vi "Autonomous Independent.vi"() -> ()   [LabVIEW 2017]
doc: "This VI is called when autonomous begins, and will automatically be terminated when autonomous ends. You can carry out timed or sensor driven robot movement independently without needing to return to the caller."
uses:
  Public/Documents/Cross The Road Electronics/Phoenix-LabVIEW/Motor Controller/Controls/CTRE_Phoenix_MotorControl_ControlMode.ctl
  <vilib>/Rock Robotics/Network Tables/NT Read String.vi
  <vilib>/Rock Robotics/Network Tables/NT Read Number.vi
  <vilib>/Rock Robotics/Network Tables/NT Read Numeric Array.vi
  <vilib>/Rock Robotics/Network Tables/NT Read String Array.vi
  Robot Global Data.vi
  <vilib>/Rock Robotics/WPI/Ultrasonic/WPI_SonarMB1010AnalogRefNum Registry Get.vi
  <vilib>/Rock Robotics/WPI/Ultrasonic/WPI_SonarMB1010AnalogGetRange.vi
panel:
  out "Setpoint2":dbl
  out "Setpoint":dbl
  in  "Z Drive PID Gains":T1={"Position"=0.04, "Interval"=0.0, "Derivative"=0.0}
  # "Be sure to right-click and choose Data Operations>>Make Current Value default if you want to save the array values with the VI"
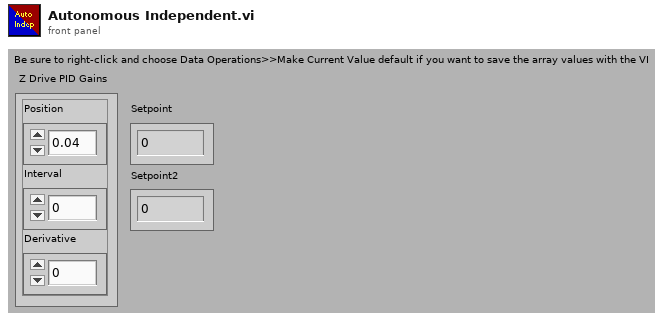
[diagram p1: front panel]
types:
  T1 = cluster{"Position":dbl, "Interval":dbl, "Derivative":dbl}
  T2 = enum16{"Front Left", "Front Right", "Back Left", "Back Right"}
  T3 = typedef "WPI_SonarMB1010AnalogDeviceRef.ctl" = cluster{"AIDeviceRef":T4, "Scaling factor (V/in)":dbl, "Average Bits":u8}
  T4 = typedef "WPI_AnalogChannelDevRef.ctl" = cluster{"DevStatus":errorcluster, "Analog Channel":T5}
  T5 = typedef "FPGA_AIChannel.ctl" = enum8{"AI 0", "AI 1", "AI 2", "AI 3", "AI MXP 0", "AI MXP 1", "AI MXP 2", "AI MXP 3", "Invalid"}
  T6 = typedef "WPI_AccelerometerDevRef.ctl" = cluster{"DevStatus":errorcluster, "Scaling":T7, "Analog Channels":T8, "I2C Bus":T9, "SPI Bus":T10, "Accel Range":T11, "ADXL Axes":T12, "Handle":i32, "Device Address":u8, "Accel Type":enum16{"Analog", "ADXL345 I2C", "ADXL345 SPI", "Internal", "ADXL362 SPI"}}
  T7 = typedef "WPI_AccelerometerScaling.ctl" = cluster{"Gain (VoltsPerG)":dbl, "Center Voltage":dbl}
  T8 = typedef "WPI_AccelerometerAnalogChannels.ctl" = cluster{"X-Axis":T5, "Y-Axis":T5, "Z-Axis":T5}
  T9 = typedef "i2c_bus.ctl" = enum16{"I2C On-Board", "I2C MXP", "Invalid"}
  T10 = typedef "spi_bus.ctl" = enum16{"SPI On-Board, CS0", "SPI On-Board, CS1", "SPI On-Board, CS2", "SPI On-Board, CS3", "SPI MXP", "Invalid"}
  T11 = typedef "ADXL345 Range.ctl" = u8
  T12 = typedef "WPI_AccelerometerADXL345 Axes.ctl" = cluster{"X-Axis":bool, "Y-Axis":bool, "Z-Axis":bool}
  T13 = cluster{"X-Axis":dbl, "Y-Axis":dbl, "Z-Axis":dbl}
  T14 = typedef "WPI_EncoderDevRef.ctl" = cluster{"DevStatus":errorcluster, "EncoderIndex":T15, "CounterIndex":T16, "DistancePerCount":dbl, "Decoding Type":T17}
  T15 = typedef "FPGA_EncoderIdx.ctl" = enum8{"Enc 0", "Enc 1", "Enc 2", "Enc 3", "Enc 4", "Enc 5", "Enc 6", "Enc 7", "Invalid"}
  T16 = typedef "FPGA_CounterCtrSystemIndex.ctl" = enum8{"Ctr 0", "Ctr 1", "Ctr 2", "Ctr 3", "Ctr 4", "Ctr 5", "Ctr 6", "Ctr 7", "Invalid"}
  T17 = typedef "WPI_EncoderType.ctl" = enum16{"1x", "2x", "4x"}
  T18 = typedef "WPI_MotorControlDeviceRef.ctl" = cluster{"DeviceStatus":errorcluster, "Type":T19, "PWM":cluster{"PWM Channel":T20, "DeadBand":T21}, "CAN":cluster{"Device Number":u8, "SetOutput VI Ref":variant, "GetOutput VI Ref":variant, "Enable VI Ref":variant, "Disable VI Ref":variant, "Data":variant}, "Invert":bool, "DIO PWM":cluster{"PWM \"Enable\" Channel":T20, "DIOChannel":T22, "PWM Rate":dbl}}
  T19 = typedef "WPI_MotorControlType.ctl" = enum16{"PWM", "CAN", "DIO PWM"}
  T20 = typedef "FPGA_DIOPWMChannel.ctl" = enum8{"PWM 0", "PWM 1", "PWM 2", "PWM 3", "PWM 4", "PWM 5", "PWM 6", "PWM 7", "PWM 8", "PWM 9", "PWM MXP 0", "PWM MXP 1", "PWM MXP 2", "PWM MXP 3", "PWM MXP 4", "PWM MXP 5", "PWM MXP 6", "PWM MXP 7", "PWM MXP 8", "PWM MXP 9", "Invalid"}
  T21 = typedef "WPI_PWMDeadband.ctl" = cluster{"Name":string, "maxPositivePwm":i32, "minPositivePwm":i32, "centerPwm":i32, "maxNegativePwm":i32, "minNegativePwm":i32, "angularRange":u16}
  T22 = typedef "FPGA_DIOChannel.ctl" = enum8{"DIO 0", "DIO 1", "DIO 2", "DIO 3", "DIO 4", "DIO 5", "DIO 6", "DIO 7", "DIO 8", "DIO 9", "DIO MXP 0", "DIO MXP 1", "DIO MXP 2", "DIO MXP 3", "DIO MXP 4", "DIO MXP 5", "DIO MXP 6", "DIO MXP 7", "DIO MXP 8", "DIO MXP 9", "DIO MXP 10", "DIO MXP 11", "DIO MXP 12", "DIO MXP 13", "DIO MXP 14", "DIO MXP 15", "SPI Port CS1", "SPI Port CS2", "SPI Port CS3", "SPI Port MISO", "SPI Port MOSI", "Invalid"}
  T23 = typedef "CTRE_Phoenix_MotorControl_ControlMode.ctl" = u16
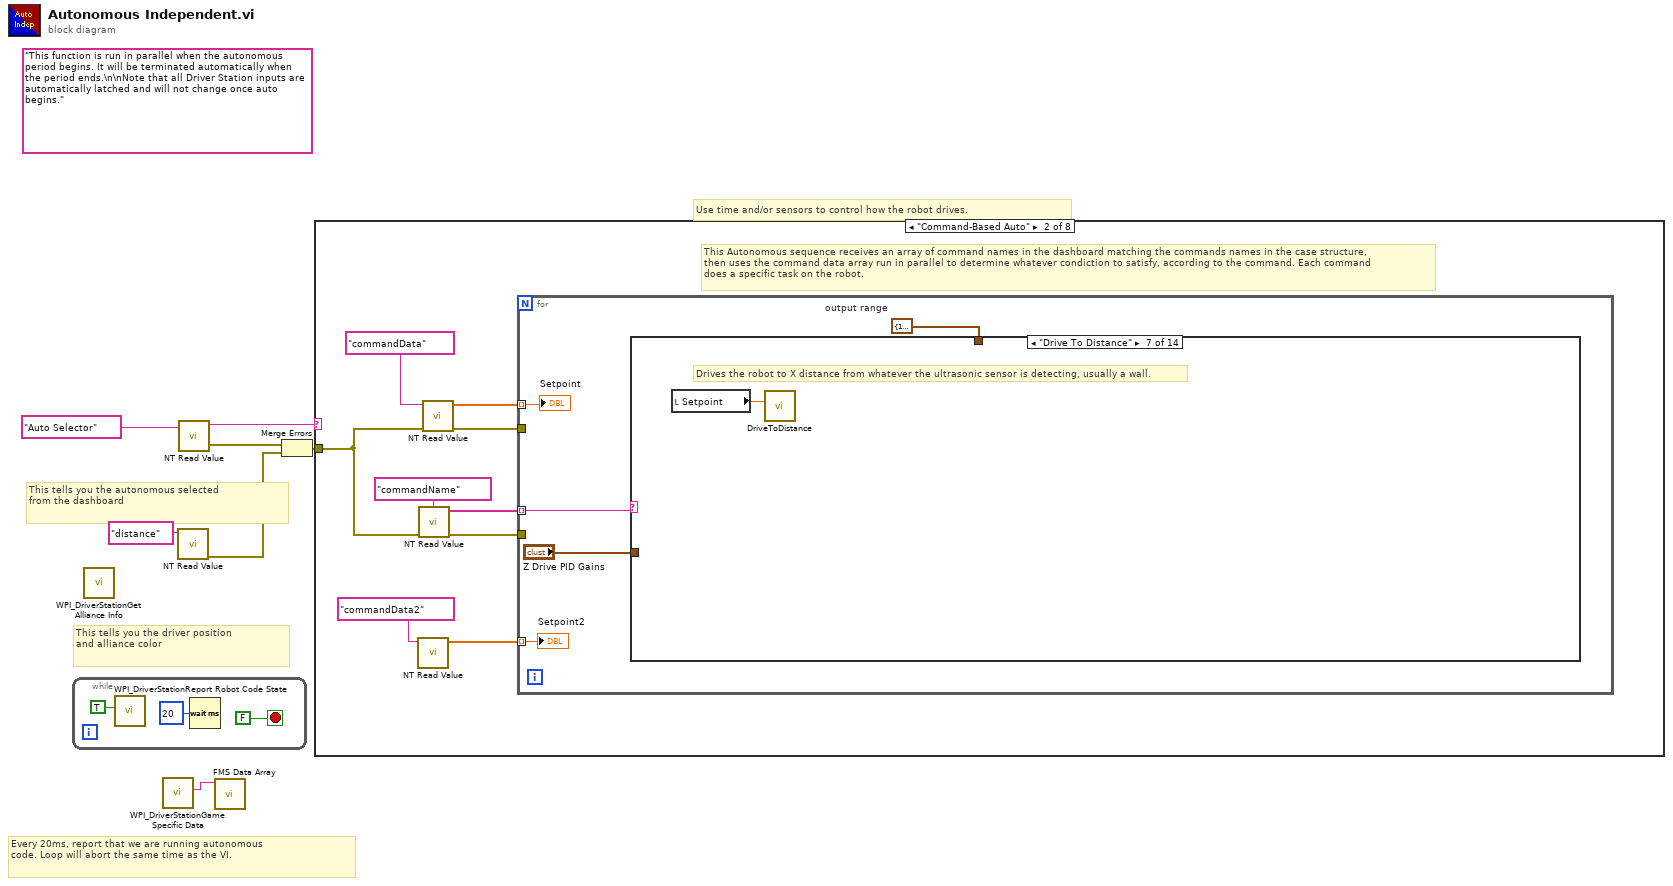
[diagram p0: block diagram]
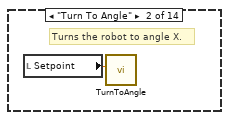
[diagram p4: hidden frame]
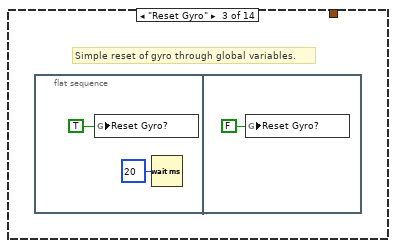
[diagram p5: hidden frame]
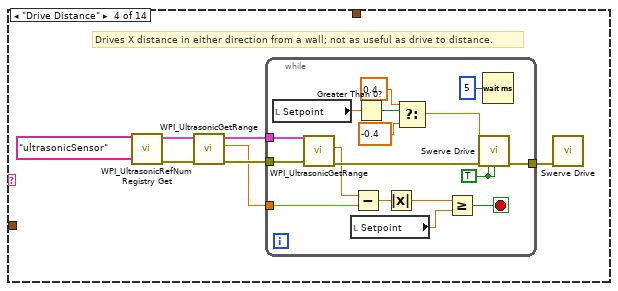
[diagram p6: hidden frame]
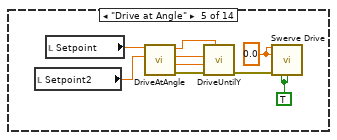
[diagram p7: hidden frame]
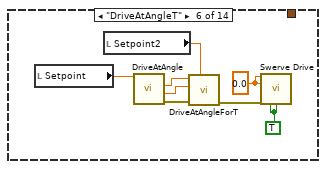
[diagram p8: hidden frame]
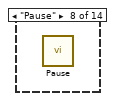
[diagram p9: hidden frame]
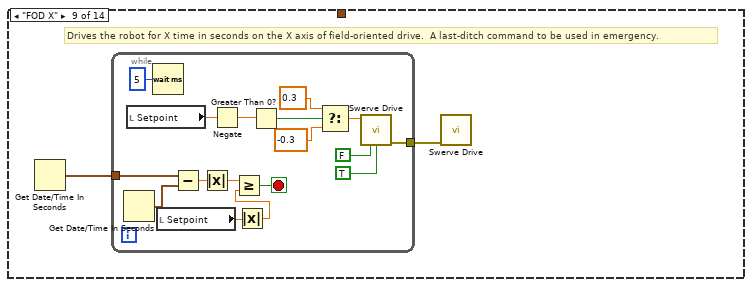
[diagram p10: hidden frame]
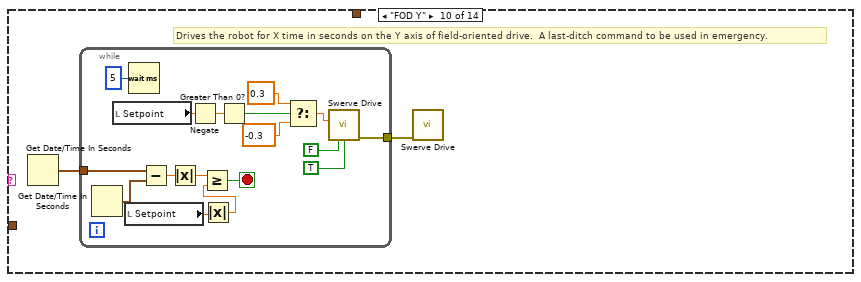
[diagram p11: hidden frame]
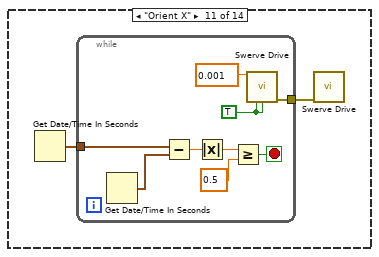
[diagram p12: hidden frame]
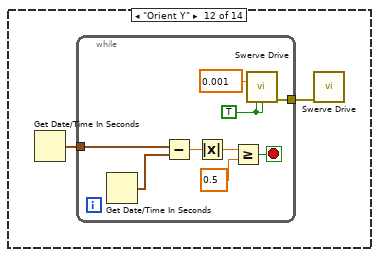
[diagram p13: hidden frame]
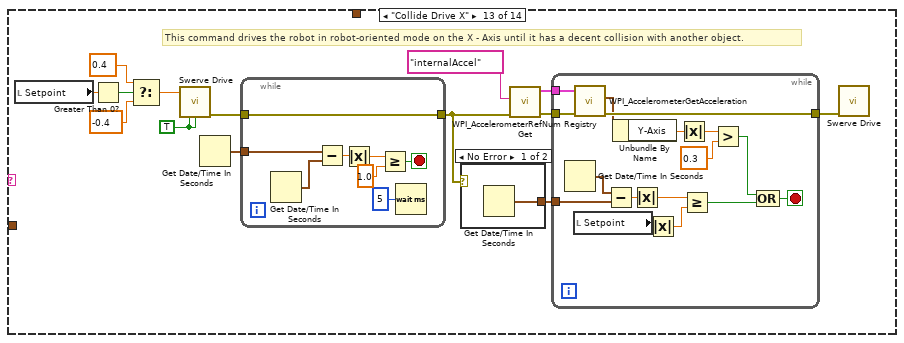
[diagram p14: hidden frame]
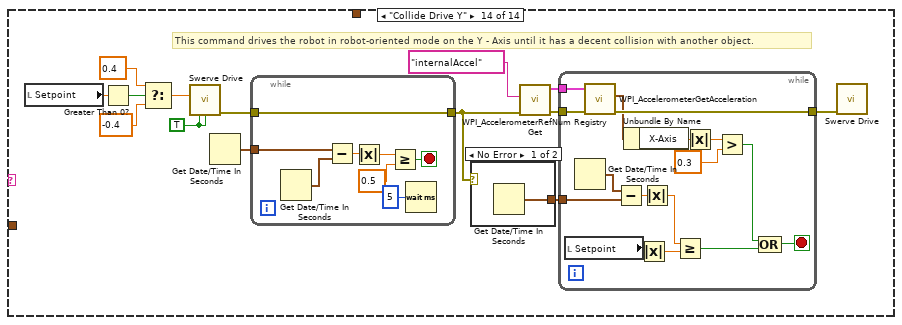
[diagram p16: hidden frame]
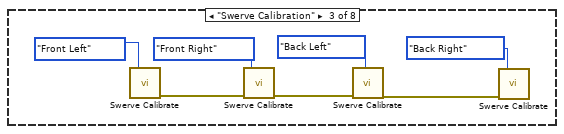
[diagram p18: hidden frame]
diagram:
  (unwired) "This function is run in parallel when the autonomous period begins. It will be terminated automatically when the period ends.\n\nNote that all Driver Station inputs are automatically latched and will not change once auto begins."
  # "This tells you the autonomous selected\nfrom the dashboard"
  # "Every 20ms, report that we are running autonomous\ncode. Loop will abort the same time as the VI."
  # "Use time and/or sensors to control how the robot drives."
  # "This tells you the driver position\nand alliance color"
  n1 = while {
    stop <- FALSE stop-if-true
    n2 = call <vilib>:"WPI_DriverStationReport Robot Code State.vi"("Autonomous"=TRUE) -> ()  [unwired: 10 in, 1 out]
    n3 = Wait (ms)(milliseconds to wait=u32 20) -> ()  [unwired: 1 out]
  }
  n4 = call <vilib>:"WPI_DriverStationGet Alliance Info.vi"() -> ()  [unwired: 12 out]
  n5 = call <vilib>:"WPI_DriverStationGame Specific Data.vi"() -> ("Game Specific Data"=w1:string)  [unwired: 11 in]
  n6 = call-poly <vilib>:"NT Read Value.vi"("Name"="distance") -> ("error out"=w3:errorcluster)  [unwired: 9 in, 1 out]
  n7 = call-poly <vilib>:"NT Read Value.vi"("Name"="Auto Selector") -> ("error out"=w4:errorcluster, "String"=w6:string)  [unwired: 9 in]
  n8 = call "FMS Data Array.vi"("Game Data"=w1) -> ()  [unwired: 8 in, 3 out]
  n9 = Merge Errors(w4, w3) -> (w2:errorcluster)
  n10 = case shown="\"Command-Based Auto\"" w6 {
    tunnel: w2 -> [_ w13 _ _ _ _ _ _]
    frame Default {
      # "You can put your main auto here, or you can right-click on the case and make any\nother frame be the default case."
      # "This is the frame that will execute if no selection is made, or if it is not recognized"
    }
    frame "Command-Based Auto" {
      # "This Autonomous sequence receives an array of command names in the dashboard matching the commands names in the case structure, \nthen uses the command data array run in parallel to determine whatever condiction to satisfy, according to the command. Each command\ndoes a specific task on the robot."
      n11 = call-poly <vilib>:"NT Read Value.vi"("Name"="commandData2") -> ("Numeric Array"=w11:dbl[])  [unwired: 9 in, 1 out]
      n12 = call-poly <vilib>:"NT Read Value.vi"("error in"=w13, "Name"="commandName") -> ("error out"=w14:errorcluster, "String Array"=w17:string[])  [unwired: 8 in]
      n13 = call-poly <vilib>:"NT Read Value.vi"("error in"=w13, "Name"="commandData") -> ("error out"=w15:errorcluster, "Numeric Array"=w16:dbl[])  [unwired: 8 in]
      n14 = for {
        tunnel: w17 -> [w24] mode=indexing
        tunnel: w16 -> [w21] mode=indexing
        tunnel: w15 -> [_]
        tunnel: w14 -> [_]
        tunnel: w11 -> [w20] mode=indexing
        w22 = cluster{"output high":dbl, "output low":dbl} {"output high"=1.0, "output low"=-1.0}  # output range
        n15 = case shown="\"Drive To Distance\"" w24 {
          tunnel: "Z Drive PID Gains" -> [_ _ _ _ _ _ _ _ _ _ _ _ _ _]
          tunnel: w22 -> [_ _ _ _ _ _ _ _ _ _ _ _ _ _]
          frame Default {
          }
          frame "Turn To Angle" {
            # "Turns the robot to angle X."
            n16 = local read "Setpoint"() -> (w25:dbl)
            n17 = call "TurnToAngle.vi"("Target Angle"=w25) -> ()  [unwired: 10 in, 1 out]
          }
          frame "Reset Gyro" {
            # "Simple reset of gyro through global variables."
            n18 = flat-sequence {
              frame #0 {
                n19 = global write "Robot Global Data.vi" "Reset Gyro?"(TRUE ("Reset Gyro?")) -> ()
                n20 = Wait (ms)(milliseconds to wait=u32 20) -> ()  [unwired: 1 out]
              }
              frame #1 {
                n21 = global write "Robot Global Data.vi" "Reset Gyro?"(FALSE ("Reset Gyro?")) -> ()
              }
            }
          }
          frame "Drive Distance" {
            # "Drives X distance in either direction from a wall; not as useful as drive to distance."
            n22 = call-poly <vilib>:"WPI_UltrasonicRefNum Registry Get.vi"("refnum name"="ultrasonicSensor") -> ("error out"=w31:errorcluster, "SonarMB1010AnalogDevRef"=w33:T3)  [unwired: 9 in]
            n23 = call-poly <vilib>:"WPI_UltrasonicGetRange.vi"("error in"=w31, "SonarMB1010AnalogDevRef"=w33) -> ("error out"=w30:errorcluster, "Distance"=w29:dbl, "SonarMB1010AnalogDevRef"=w32:T3)  [unwired: 7 in]
            n24 = while {
              tunnel: [w51] -> w34
              tunnel: w29 -> [w46]
              tunnel: w32 -> [w49]
              tunnel: w30 -> [w48]
              stop <- w50 stop-if-true
              w41 = TRUE ("Robot Centric?")
              n25 = local read "Setpoint"() -> (w39:dbl)
              n26 = call-poly <vilib>:"WPI_UltrasonicGetRange.vi"("error in"=w48, "SonarMB1010AnalogDevRef"=w49) -> ("error out"=w47:errorcluster, "Distance"=w40:dbl)  [unwired: 7 in, 1 out]
              n27 = local read "Setpoint"() -> (w38:dbl)
              n28 = Subtract(x=w40, y=w46) -> (x-y=w37:dbl)
              n29 = Greater Than 0?(x=w39) -> (x > 0?=w42:bool)
              n30 = Absolute Value(x=w37) -> (abs(x)=w52:dbl)
              n31 = Select(t=0.4 ("Y"), s=w42, f=-0.4 ("Y")) -> (s? t:f=w45:dbl)
              n32 = Greater Or Equal?(x=w52, y=w38) -> (x >= y?=w50:bool)
              n33 = call "Swerve Drive.vi"("Y"=w45, "Error In"=w47, "Robot Centric?"=w41, "Autonomous?"=w41) -> ("Error Out"=w51:errorcluster)  [unwired: 7 in, 4 out]
              n34 = Wait (ms)(milliseconds to wait=u32 5) -> ()  [unwired: 1 out]
            }
            n35 = call "Swerve Drive.vi"("Error In"=w34) -> ()  [unwired: 10 in, 5 out]
          }
          frame "Drive at Angle" {
            w56 = TRUE ("Autonomous?")
            w57 = 0.0
            n36 = local read "Setpoint2"() -> (w53:dbl)
            n37 = local read "Setpoint"() -> (w54:dbl)
            n38 = call "DriveAtAngle.vi"("Target Angle"=w54, "Distance"=w53) -> ("y-axis distance"=w55:dbl, "x"=w59:dbl, "y"=w58:dbl, "Error Out"=w60:errorcluster)  [unwired: 5 in]
            n39 = call "DriveUntilY.vi"("Ultrasonic Stop"=w55, "error in"=w60, "y"=w58, "x"=w59) -> ("error out"=w61:errorcluster)  [unwired: 7 in]
            n40 = call "Swerve Drive.vi"("X"=w57, "Y"=w57, "Error In"=w61, "Robot Centric?"=w56, "Autonomous?"=w56) -> ()  [unwired: 6 in, 5 out]
          }
          frame "DriveAtAngleT" {
            w67 = TRUE ("Autonomous?")
            w68 = 0.0
            n41 = local read "Setpoint"() -> (w69:dbl)
            n42 = local read "Setpoint2"() -> (w62:dbl)
            n43 = call "DriveAtAngle.vi"("Target Angle"=w69) -> ("x"=w66:dbl, "y"=w65:dbl, "Error Out"=w64:errorcluster)  [unwired: 6 in, 1 out]
            n44 = call "DriveAtAngleForT.vi"("time(sec)"=w62, "Error In"=w64, "y"=w65, "x"=w66) -> ("Error Out"=w63:errorcluster)  [unwired: 7 in]
            n45 = call "Swerve Drive.vi"("X"=w68, "Y"=w68, "Error In"=w63, "Robot Centric?"=w67, "Autonomous?"=w67) -> ()  [unwired: 6 in, 5 out]
          }
          frame "Drive To Distance" {
            # "Drives the robot to X distance from whatever the ultrasonic sensor is detecting, usually a wall."
            n46 = local read "Setpoint"() -> (w70:dbl)
            n47 = call "DriveToDistance.vi"("Setpoint"=w70) -> ()  [unwired: 10 in, 1 out]
          }
          frame "Pause" {
            n48 = call "Pause.vi"() -> ()  [unwired: 11 in, 1 out]
          }
          frame "FOD X" {
            # "Drives the robot for X time in seconds on the X axis of field-oriented drive.  A last-ditch command to be used in emergency."
            n49 = Get Date/Time In Seconds() -> (seconds since 1Jan1904=w72:timestamp)
            n50 = while {
              tunnel: w72 -> [w89]
              tunnel: [w83] -> w71
              stop <- w84 stop-if-true
              n51 = Get Date/Time In Seconds() -> (seconds since 1Jan1904=w88:timestamp)
              n52 = local read "Setpoint"() -> (w76:dbl)
              n53 = Wait (ms)(milliseconds to wait=u32 5) -> ()  [unwired: 1 out]
              n54 = local read "Setpoint"() -> (w85:dbl)
              n55 = Subtract(x=w89, y=w88) -> (x-y=w87:dbl)
              n56 = Absolute Value(x=w87) -> (abs(x)=w86:dbl)
              n57 = Negate(x=w76) -> (-x=w73:dbl)
              n58 = Absolute Value(x=w85) -> (abs(x)=w74:dbl)
              n59 = Greater Or Equal?(x=w86, y=w74) -> (x >= y?=w84:bool)
              n60 = Greater Than 0?(x=w73) -> (x > 0?=w77:bool)
              n61 = Select(t=0.3 ("X"), s=w77, f=-0.3 ("X")) -> (s? t:f=w78:dbl)
              n62 = call "Swerve Drive.vi"("X"=w78, "Robot Centric?"=FALSE, "Autonomous?"=TRUE) -> ("Error Out"=w83:errorcluster)  [unwired: 8 in, 4 out]
            }
            n63 = call "Swerve Drive.vi"("Error In"=w71) -> ()  [unwired: 10 in, 5 out]
          }
          frame "FOD Y" {
            # "Drives the robot for X time in seconds on the Y axis of field-oriented drive.  A last-ditch command to be used in emergency."
            n64 = Get Date/Time In Seconds() -> (seconds since 1Jan1904=w91:timestamp)
            n65 = while {
              tunnel: w91 -> [w108]
              tunnel: [w102] -> w90
              stop <- w103 stop-if-true
              n66 = Get Date/Time In Seconds() -> (seconds since 1Jan1904=w107:timestamp)
              n67 = local read "Setpoint"() -> (w95:dbl)
              n68 = local read "Setpoint"() -> (w104:dbl)
              n69 = Wait (ms)(milliseconds to wait=u32 5) -> ()  [unwired: 1 out]
              n70 = Subtract(x=w108, y=w107) -> (x-y=w106:dbl)
              n71 = Absolute Value(x=w106) -> (abs(x)=w105:dbl)
              n72 = Negate(x=w95) -> (-x=w92:dbl)
              n73 = Absolute Value(x=w104) -> (abs(x)=w93:dbl)
              n74 = Greater Or Equal?(x=w105, y=w93) -> (x >= y?=w103:bool)
              n75 = Greater Than 0?(x=w92) -> (x > 0?=w97:bool)
              n76 = Select(t=0.3 ("X"), s=w97, f=-0.3 ("X")) -> (s? t:f=w96:dbl)
              n77 = call "Swerve Drive.vi"("Y"=w96, "Robot Centric?"=FALSE, "Autonomous?"=TRUE) -> ("Error Out"=w102:errorcluster)  [unwired: 8 in, 4 out]
            }
            n78 = call "Swerve Drive.vi"("Error In"=w90) -> ()  [unwired: 10 in, 5 out]
          }
          frame "Orient X" {
            n79 = Get Date/Time In Seconds() -> (seconds since 1Jan1904=w110:timestamp)
            n80 = while {
              tunnel: w110 -> [w119]
              tunnel: [w113] -> w109
              stop <- w112 stop-if-true
              w114 = TRUE ("Robot Centric?")
              n81 = Get Date/Time In Seconds() -> (seconds since 1Jan1904=w118:timestamp)
              n82 = Subtract(x=w119, y=w118) -> (x-y=w117:dbl)
              n83 = Absolute Value(x=w117) -> (abs(x)=w116:dbl)
              n84 = Greater Or Equal?(x=w116, y=0.5) -> (x >= y?=w112:bool)
              n85 = call "Swerve Drive.vi"("X"=0.001 ("Y"), "Robot Centric?"=w114, "Autonomous?"=w114) -> ("Error Out"=w113:errorcluster)  [unwired: 8 in, 4 out]
            }
            n86 = call "Swerve Drive.vi"("Error In"=w109) -> ()  [unwired: 10 in, 5 out]
          }
          frame "Orient Y" {
            n87 = Get Date/Time In Seconds() -> (seconds since 1Jan1904=w121:timestamp)
            n88 = while {
              tunnel: w121 -> [w130]
              tunnel: [w123] -> w120
              stop <- w122 stop-if-true
              w125 = TRUE ("Robot Centric?")
              n89 = Get Date/Time In Seconds() -> (seconds since 1Jan1904=w129:timestamp)
              n90 = Subtract(x=w130, y=w129) -> (x-y=w128:dbl)
              n91 = Absolute Value(x=w128) -> (abs(x)=w127:dbl)
              n92 = Greater Or Equal?(x=w127, y=0.5) -> (x >= y?=w122:bool)
              n93 = call "Swerve Drive.vi"("Y"=0.001, "Robot Centric?"=w125, "Autonomous?"=w125) -> ("Error Out"=w123:errorcluster)  [unwired: 8 in, 4 out]
            }
            n94 = call "Swerve Drive.vi"("Error In"=w120) -> ()  [unwired: 10 in, 5 out]
          }
          frame "Collide Drive X" {
            w139 = TRUE ("Robot Centric?")
            # "This command drives the robot in robot-oriented mode on the X - Axis until it has a decent collision with another object."
            n95 = local read "Setpoint"() -> (w144:dbl)
            n96 = Greater Than 0?(x=w144) -> (x > 0?=w143:bool)
            n97 = Select(t=0.4, s=w143, f=-0.4) -> (s? t:f=w140:dbl)
            n98 = call "Swerve Drive.vi"("X"=w140, "Robot Centric?"=w139, "Autonomous?"=w139) -> ("Error Out"=w138:errorcluster)  [unwired: 8 in, 4 out]
            n99 = Get Date/Time In Seconds() -> (seconds since 1Jan1904=w137:timestamp)
            n100 = while {
              tunnel: w138 -> [w162]
              tunnel: w137 -> [w169]
              tunnel: [w162] -> w132
              stop <- w163 stop-if-true
              n101 = Get Date/Time In Seconds() -> (seconds since 1Jan1904=w168:timestamp)
              n102 = Subtract(x=w169, y=w168) -> (x-y=w167:dbl)
              n103 = Absolute Value(x=w167) -> (abs(x)=w166:dbl)
              n104 = Greater Or Equal?(x=w166, y=1.0) -> (x >= y?=w163:bool)
              n105 = Wait (ms)(milliseconds to wait=u32 5) -> ()  [unwired: 1 out]
            }
            n106 = case shown="No Error" w132 {
              tunnel: [w145 _] -> w131
              frame No Error {
                n107 = Get Date/Time In Seconds() -> (seconds since 1Jan1904=w145:timestamp)
              }
              frame Error {
              }
            }
            n108 = call <vilib>:"WPI_AccelerometerRefNum Registry Get.vi"("error in (no error)"=w132, "refnum name"="internalAccel") -> ("error out"=w135:errorcluster, "AccelerometerDevRef"=w134:T6)  [unwired: 8 in]
            n109 = while {
              tunnel: w135 -> [w161]
              tunnel: w134 -> [w160]
              tunnel: [w159] -> w133
              tunnel: w131 -> [w157]
              stop <- w158 stop-if-true
              n110 = Get Date/Time In Seconds() -> (seconds since 1Jan1904=w156:timestamp)
              n111 = local read "Setpoint"() -> (w152:dbl)
              n112 = call <vilib>:"WPI_AccelerometerGetAcceleration.vi"("error in"=w161, "AccelerometerDevRef"=w160) -> ("error out"=w159:errorcluster, "Accelerations"=w150:T13)  [unwired: 7 in, 1 out]
              n113 = Subtract(x=w156, y=w157) -> (x-y=w155:dbl)
              n114 = Unbundle By Name(w150) -> ("Y-Axis"=w149:dbl)
              n115 = Absolute Value(x=w155) -> (abs(x)=w154:dbl)
              n116 = Absolute Value(x=w152) -> (abs(x)=w151:dbl)
              n117 = Absolute Value(x=w149) -> (abs(x)=w147:dbl)
              n118 = Greater Or Equal?(x=w154, y=w151) -> (x >= y?=w153:bool)
              n119 = Greater?(x=w147, y=0.3) -> (0:w146:bool)
              n120 = Compound Arithmetic op=OR(w146, w153) -> (w158:bool)
            }
            n121 = call "Swerve Drive.vi"("Error In"=w133) -> ()  [unwired: 10 in, 5 out]
          }
          frame "Collide Drive Y" {
            w179 = TRUE ("Robot Centric?")
            # "This command drives the robot in robot-oriented mode on the Y - Axis until it has a decent collision with another object."
            n122 = local read "Setpoint"() -> (w183:dbl)
            n123 = Greater Than 0?(x=w183) -> (x > 0?=w182:bool)
            n124 = Select(t=0.4, s=w182, f=-0.4) -> (s? t:f=w170:dbl)
            n125 = call "Swerve Drive.vi"("Y"=w170, "Robot Centric?"=w179, "Autonomous?"=w179) -> ("Error Out"=w178:errorcluster)  [unwired: 8 in, 4 out]
            n126 = Get Date/Time In Seconds() -> (seconds since 1Jan1904=w177:timestamp)
            n127 = while {
              tunnel: w178 -> [w201]
              tunnel: w177 -> [w208]
              tunnel: [w201] -> w172
              stop <- w202 stop-if-true
              n128 = Get Date/Time In Seconds() -> (seconds since 1Jan1904=w207:timestamp)
              n129 = Subtract(x=w208, y=w207) -> (x-y=w206:dbl)
              n130 = Absolute Value(x=w206) -> (abs(x)=w205:dbl)
              n131 = Greater Or Equal?(x=w205, y=0.5) -> (x >= y?=w202:bool)
              n132 = Wait (ms)(milliseconds to wait=u32 5) -> ()  [unwired: 1 out]
            }
            n133 = case shown="No Error" w172 {
              tunnel: [w184 _] -> w171
              frame No Error {
                n134 = Get Date/Time In Seconds() -> (seconds since 1Jan1904=w184:timestamp)
              }
              frame Error {
              }
            }
            n135 = call <vilib>:"WPI_AccelerometerRefNum Registry Get.vi"("error in (no error)"=w172, "refnum name"="internalAccel") -> ("error out"=w175:errorcluster, "AccelerometerDevRef"=w174:T6)  [unwired: 8 in]
            n136 = while {
              tunnel: w175 -> [w200]
              tunnel: w174 -> [w199]
              tunnel: [w198] -> w173
              tunnel: w171 -> [w195]
              stop <- w197 stop-if-true
              n137 = local read "Setpoint"() -> (w190:dbl)
              n138 = Get Date/Time In Seconds() -> (seconds since 1Jan1904=w194:timestamp)
              n139 = call <vilib>:"WPI_AccelerometerGetAcceleration.vi"("error in"=w200, "AccelerometerDevRef"=w199) -> ("error out"=w198:errorcluster, "Accelerations"=w188:T13)  [unwired: 7 in, 1 out]
              n140 = Subtract(x=w194, y=w195) -> (x-y=w193:dbl)
              n141 = Unbundle By Name(w188) -> ("X-Axis"=w187:dbl)
              n142 = Absolute Value(x=w190) -> (abs(x)=w189:dbl)
              n143 = Absolute Value(x=w193) -> (abs(x)=w192:dbl)
              n144 = Greater Or Equal?(x=w192, y=w189) -> (x >= y?=w191:bool)
              n145 = Absolute Value(x=w187) -> (abs(x)=w186:dbl)
              n146 = Greater?(x=w186, y=0.3) -> (0:w196:bool)
              n147 = Compound Arithmetic op=OR(w196, w191) -> (w197:bool)
            }
            n148 = call "Swerve Drive.vi"("Error In"=w173) -> ()  [unwired: 10 in, 5 out]
          }
        }
        "Setpoint" <- w21
        "Setpoint2" <- w20
      }
    }
    frame "Swerve Calibration" {
      n149 = call "Swerve Calibrate.vi"("Wheel Corner"=T2."Front Left") -> ("error out"=w211:errorcluster)  [unwired: 10 in]
      n150 = call "Swerve Calibrate.vi"("error in (no error)"=w211, "Wheel Corner"=T2."Front Right") -> ("error out"=w210:errorcluster)  [unwired: 9 in]
      n151 = call "Swerve Calibrate.vi"("error in (no error)"=w210, "Wheel Corner"=T2."Back Left") -> ("error out"=w209:errorcluster)  [unwired: 9 in]
      n152 = call "Swerve Calibrate.vi"("error in (no error)"=w209, "Wheel Corner"=T2."Back Right") -> ()  [unwired: 9 in, 1 out]
    }
    frame "Config 1" {
    }
    frame "Config 2" {
    }
    frame "Config 3" {
    }
    frame "Motor Jog Mode" {
    }
    frame "Unwind Motors" {
      n153 = call <vilib>:"WPI_EncoderRefNum Registry Get.vi"("refnum name"="frontRightEnc") -> ("error out"=w242:errorcluster, "EncoderDevRef"=w241:T14)  [unwired: 9 in]
      n154 = call <vilib>:"WPI_EncoderRefNum Registry Get.vi"("refnum name"="frontLeftEnc") -> ("error out"=w249:errorcluster, "EncoderDevRef"=w250:T14)  [unwired: 9 in]
      n155 = call "CTRE_Phoenix_MotorControl_RefNumRegistryGet.vi"("refnum name"="frontLeftRotation") -> ("error out"=w225:errorcluster, "PhoenixMotorControlDevRef"=w226:T18)  [unwired: 9 in]
      n156 = call "CTRE_Phoenix_MotorControl_RefNumRegistryGet.vi"("refnum name"="frontRightRotation") -> ("error out"=w223:errorcluster, "PhoenixMotorControlDevRef"=w224:T18)  [unwired: 9 in]
      n157 = call <vilib>:"WPI_EncoderGet.vi"("error in (no error)"=w242, "EncoderDevRef"=w241) -> ("error out"=w243:errorcluster, "Distance"=w245:dbl, "EncoderDevRef"=w244:T14)  [unwired: 4 in, 3 out]
      n158 = call <vilib>:"WPI_EncoderGet.vi"("error in (no error)"=w249, "EncoderDevRef"=w250) -> ("error out"=w248:errorcluster, "Distance"=w246:dbl, "EncoderDevRef"=w247:T14)  [unwired: 4 in, 3 out]
      n159 = while {
        tunnel: w244 -> [w296]
        tunnel: w243 -> [w295]
        tunnel: w245 -> [w294]
        tunnel: w224 -> [w283]
        tunnel: w223 -> [w285]
        stop <- w289 stop-if-true
        w282 = T23 0 items=["PercentOutput"=0, "Position"=1, "Velocity"=2, "Current"=3, "Follower"=5, "MotionProfile"=6, "MotionMagic"=7, "MotionMagicArc"=8, "MotionProfileArc"=10, "Disabled"=15] ("Control Mode")
        n160 = Greater Than 0?(x=w294) -> (x > 0?=w293:bool)
        n161 = call <vilib>:"WPI_EncoderGet.vi"("error in (no error)"=w295, "EncoderDevRef"=w296) -> ("Distance"=w288:dbl)  [unwired: 4 in, 5 out]
        n162 = Select(t=0.5, s=w293, f=-0.5) -> (s? t:f=w284:dbl)
        n163 = In Range and Coerce(upper limit=1.0, x=w288, lower limit=-1.0) -> (In Range?=w289:bool)  [unwired: 1 out]
        n164 = call "CTRE_Phoenix_MotorControl_Set.vi"("error in (no error)"=w285, "Output"=w284, "Control Mode"=w282, "PhoenixMotorControlDevRef"=w283) -> ()  [unwired: 5 in, 3 out]
        n165 = Wait (ms)(milliseconds to wait=u32 5) -> ()  [unwired: 1 out]
      }
      n166 = while {
        tunnel: w247 -> [w311]
        tunnel: w248 -> [w310]
        tunnel: w246 -> [w309]
        tunnel: w226 -> [w300]
        tunnel: w225 -> [w299]
        stop <- w304 stop-if-true
        w297 = T23 0 items=["PercentOutput"=0, "Position"=1, "Velocity"=2, "Current"=3, "Follower"=5, "MotionProfile"=6, "MotionMagic"=7, "MotionMagicArc"=8, "MotionProfileArc"=10, "Disabled"=15] ("Control Mode")
        n167 = Greater Than 0?(x=w309) -> (x > 0?=w308:bool)
        n168 = call <vilib>:"WPI_EncoderGet.vi"("error in (no error)"=w310, "EncoderDevRef"=w311) -> ("Distance"=w303:dbl)  [unwired: 4 in, 5 out]
        n169 = Select(t=0.5, s=w308, f=-0.5) -> (s? t:f=w298:dbl)
        n170 = In Range and Coerce(upper limit=1.0, x=w303, lower limit=-1.0) -> (In Range?=w304:bool)  [unwired: 1 out]
        n171 = call "CTRE_Phoenix_MotorControl_Set.vi"("error in (no error)"=w299, "Output"=w298, "Control Mode"=w297, "PhoenixMotorControlDevRef"=w300) -> ()  [unwired: 5 in, 3 out]
        n172 = Wait (ms)(milliseconds to wait=u32 5) -> ()  [unwired: 1 out]
      }
      n173 = call <vilib>:"WPI_EncoderRefNum Registry Get.vi"("refnum name"="backRightEnc") -> ("error out"=w230:errorcluster, "EncoderDevRef"=w229:T14)  [unwired: 9 in]
      n174 = call <vilib>:"WPI_EncoderRefNum Registry Get.vi"("refnum name"="backLeftEnc") -> ("error out"=w237:errorcluster, "EncoderDevRef"=w238:T14)  [unwired: 9 in]
      n175 = call "CTRE_Phoenix_MotorControl_RefNumRegistryGet.vi"("refnum name"="backRightRotation") -> ("error out"=w220:errorcluster, "PhoenixMotorControlDevRef"=w221:T18)  [unwired: 9 in]
      n176 = call "CTRE_Phoenix_MotorControl_RefNumRegistryGet.vi"("refnum name"="backLeftRotation") -> ("error out"=w218:errorcluster, "PhoenixMotorControlDevRef"=w217:T18)  [unwired: 9 in]
      n177 = call <vilib>:"WPI_EncoderGet.vi"("error in (no error)"=w230, "EncoderDevRef"=w229) -> ("error out"=w231:errorcluster, "Distance"=w233:dbl, "EncoderDevRef"=w232:T14)  [unwired: 4 in, 3 out]
      n178 = call <vilib>:"WPI_EncoderGet.vi"("error in (no error)"=w237, "EncoderDevRef"=w238) -> ("error out"=w236:errorcluster, "Distance"=w234:dbl, "EncoderDevRef"=w235:T14)  [unwired: 4 in, 3 out]
      n179 = while {
        tunnel: w232 -> [w266]
        tunnel: w231 -> [w265]
        tunnel: w233 -> [w264]
        tunnel: w221 -> [w255]
        tunnel: w220 -> [w253]
        stop <- w259 stop-if-true
        w252 = T23 0 items=["PercentOutput"=0, "Position"=1, "Velocity"=2, "Current"=3, "Follower"=5, "MotionProfile"=6, "MotionMagic"=7, "MotionMagicArc"=8, "MotionProfileArc"=10, "Disabled"=15] ("Control Mode")
        n180 = Greater Than 0?(x=w264) -> (x > 0?=w263:bool)
        n181 = call <vilib>:"WPI_EncoderGet.vi"("error in (no error)"=w265, "EncoderDevRef"=w266) -> ("Distance"=w258:dbl)  [unwired: 4 in, 5 out]
        n182 = Select(t=0.5, s=w263, f=-0.5) -> (s? t:f=w254:dbl)
        n183 = In Range and Coerce(upper limit=1.0, x=w258, lower limit=-1.0) -> (In Range?=w259:bool)  [unwired: 1 out]
        n184 = call "CTRE_Phoenix_MotorControl_Set.vi"("error in (no error)"=w253, "Output"=w254, "Control Mode"=w252, "PhoenixMotorControlDevRef"=w255) -> ()  [unwired: 5 in, 3 out]
        n185 = Wait (ms)(milliseconds to wait=u32 5) -> ()  [unwired: 1 out]
      }
      n186 = while {
        tunnel: w235 -> [w281]
        tunnel: w236 -> [w280]
        tunnel: w234 -> [w279]
        tunnel: w217 -> [w268]
        tunnel: w218 -> [w270]
        stop <- w274 stop-if-true
        w267 = T23 0 items=["PercentOutput"=0, "Position"=1, "Velocity"=2, "Current"=3, "Follower"=5, "MotionProfile"=6, "MotionMagic"=7, "MotionMagicArc"=8, "MotionProfileArc"=10, "Disabled"=15] ("Control Mode")
        n187 = Greater Than 0?(x=w279) -> (x > 0?=w278:bool)
        n188 = call <vilib>:"WPI_EncoderGet.vi"("error in (no error)"=w280, "EncoderDevRef"=w281) -> ("Distance"=w273:dbl)  [unwired: 4 in, 5 out]
        n189 = Select(t=0.5, s=w278, f=-0.5) -> (s? t:f=w269:dbl)
        n190 = In Range and Coerce(upper limit=1.0, x=w273, lower limit=-1.0) -> (In Range?=w274:bool)  [unwired: 1 out]
        n191 = call "CTRE_Phoenix_MotorControl_Set.vi"("error in (no error)"=w270, "Output"=w269, "Control Mode"=w267, "PhoenixMotorControlDevRef"=w268) -> ()  [unwired: 5 in, 3 out]
        n192 = Wait (ms)(milliseconds to wait=u32 5) -> ()  [unwired: 1 out]
      }
    }
  }
